vi "keccak.remain.helper.0.7.vi"(9 "HT_DATA.Valid":bool, 10 "HT_DATA.Data":u64, 11 "Variables":T2={"hash.input_size"=0, "hash.bits"=0, "state.next"=enum."Wait.for.Start", "state.after_next"=enum."Wait.for.Start", "read.i"=0, "read.block_i"=0, "hash.block_words"=0, "hash.block_size"=0, "keccak.i"=0, "state[25]"=[0, 0, 0, 0, 0, 0, 0, 0, 0, 0, 0, 0, 0, 0, 0, 0, 0, 0, 0, 0, 0, 0, 0, 0, 0], "HT_PARMS.Valid"=FALSE, "HT_PARMS.Data"=0, "Read.HT_PARMS"=FALSE, "HT_DATA.Valid"=FALSE, "HT_DATA.Data"=0, "Read.HT_DATA"=FALSE, "TH_RESULTS.Valid"=FALSE, "TH_RESULTS.Data"=0, "TH_RESULTS.Ready"=FALSE}) -> (0 "state.next":T1=enum."Keccak", 1 "state[25] out":u64[](array[numeric]), 2 "Continue?":bool, 3 "Valid":bool)   [LabVIEW 2021]
uses:
  Users/johns/OneDrive/Documents/LabVIEW Data/Untitled Project 2/CLIP/keccak.variables.ctl
  Users/johns/OneDrive/Documents/LabVIEW Data/Untitled Project 2/CLIP/keccak.states.ctl
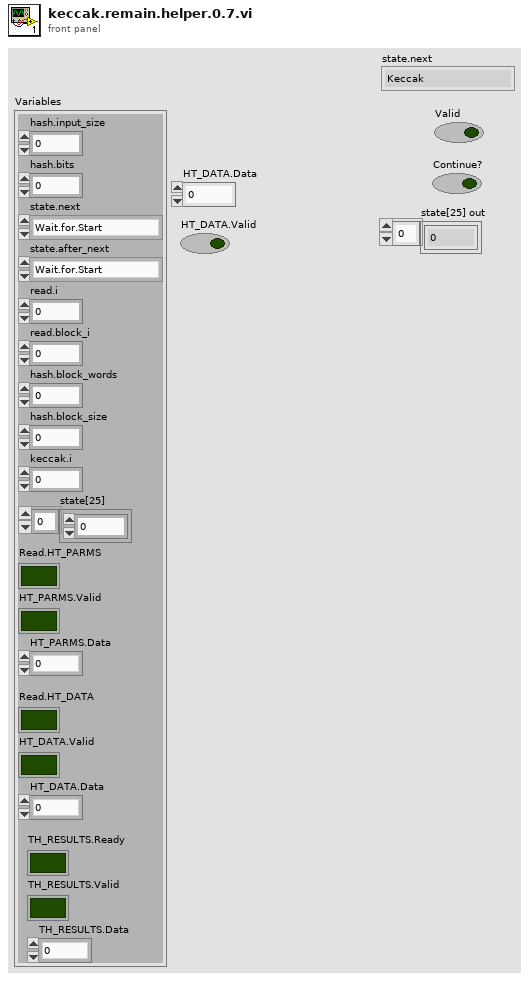
[diagram p1: front panel]
types:
  T1 = typedef "keccak.states.ctl" = enum8{"Wait.for.Start", "Read.Blocks", "Read.Remainder", "Keccak", "Send.Result"}
  T2 = typedef "keccak.variables.ctl" = cluster{"hash.input_size":u16, "hash.bits":u16, "state.next":T1, "state.after_next":T1, "read.i":u16, "read.block_i":u16, "hash.block_words":u16, "hash.block_size":u16, "keccak.i":u16, "state[25]":u64[], "HT_PARMS.Valid":bool, "HT_PARMS.Data":u64, "Read.HT_PARMS":bool, "HT_DATA.Valid":bool, "HT_DATA.Data":u64, "Read.HT_DATA":bool, "TH_RESULTS.Valid":bool, "TH_RESULTS.Data":u64, "TH_RESULTS.Ready":bool}
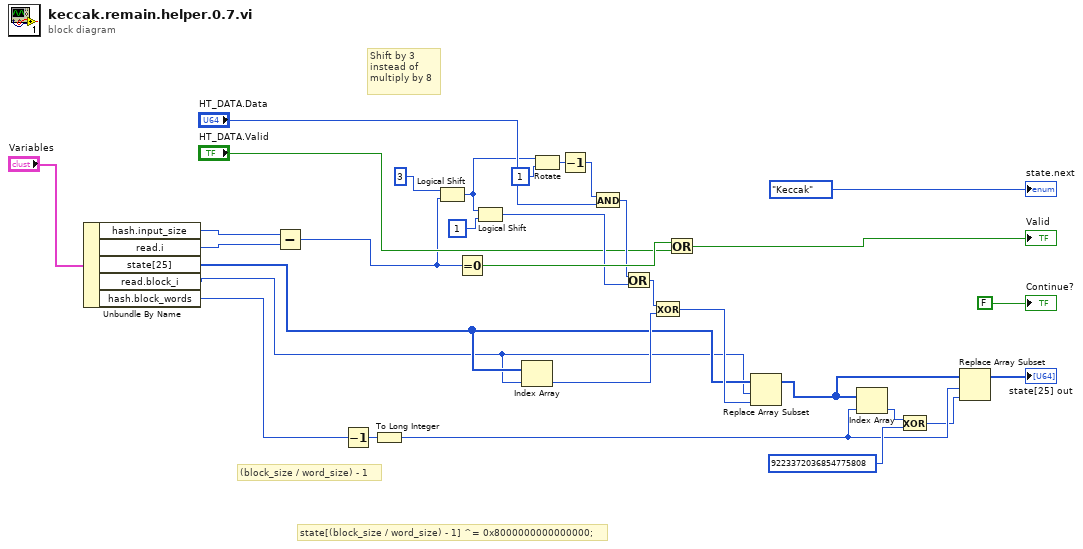
[diagram p0: block diagram]
diagram:
  # "Shift by 3\ninstead of\nmultiply by 8"
  # "state[(block_size / word_size) - 1] ^= 0x8000000000000000;"
  # "(block_size / word_size) - 1"
  n1 = Unbundle By Name("Variables") -> ("hash.input_size"=w13:u16, "read.i"=w12:u16, "state[25]"=w10:u64[], "read.block_i"=w7:u16, "hash.block_words"=w8:u16)
  n2 = Subtract(x=w13, y=w12) -> (x-y=w11:u16)
  n3 = Decrement(x=w8) -> (x-1=w16:u16)
  n4 = To Long Integer(number=w16) -> (32bit integer=w4:i32)
  n5 = Logical Shift(y=i16 3, x=w11) -> (x << y=w26:u16)
  n6 = Equal To 0?(x=w11) -> (x = 0?=w31:bool)
  n7 = Logical Shift(y=w26, x=u64 1) -> (x << y=w29:u64)
  n8 = Index Array(array=w10, index=w7) -> (element=w17:u64)
  n9 = Rotate(1:u64 1 ("x rotated left by y"), 2:w26) -> (0:w24:u64)
  n10 = Decrement(x=w24) -> (x-1=w27:u64)
  n11 = And(x=w27, y="HT_DATA.Data") -> (x .and. y?=w30:u64)
  n12 = Or(x=w30, y=w29) -> (x .or. y?=w20:u64)
  n13 = Exclusive Or(1:w17, 2:w20) -> (0:w18:u64)
  n14 = Or(x=w31, y="HT_DATA.Valid") -> (x .or. y?=→"Valid":bool)
  n15 = Replace Array Subset(array=w10, new element=w18, index=w7) -> (w5:u64[])
  n16 = Index Array(array=w5, index=w4) -> (element=w3:u64)
  n17 = Exclusive Or(1:u64 9223372036854775808, 2:w3) -> (0:w2:u64)
  n18 = Replace Array Subset(array=w5, new element=w2, index=w4) -> (→"state[25] out":u64[])
  "Continue?" <- FALSE ("Continue?")
  "state.next" <- keccak.states."Keccak" ("state.next")
